vi "GenerateCode.vi"(1 "Terms":T1[](array[typedef]), 3 "Diagram":refnum<vi>, 5 "XRef":refnum<vi>, 6 "State In":T4) -> (0 "Generated Code?":bool, 2 "State Out":T4, 4 "Reply":string[](array[string]))   [LabVIEW 2012, in "Shuffle Array.xnode"]
uses:
  Shuffle Array.xnode
  State.ctl
  <vilib>/XNodeSupport/XNodeTermIDPair.ctl
  <vilib>/XNodeSupport/XNodeTermRef.ctl
  <vilib>/XNodeSupport/XNodeString.ctl
  <vilib>/Utility/miscctls.llb/LVPositionTypeDef.ctl
  <userlib>/_LAVAcr/Scripting Tools/Scripting Tools.lvlib
  <vilib>/XNodeSupport/NI_XNodeSupport.lvlib
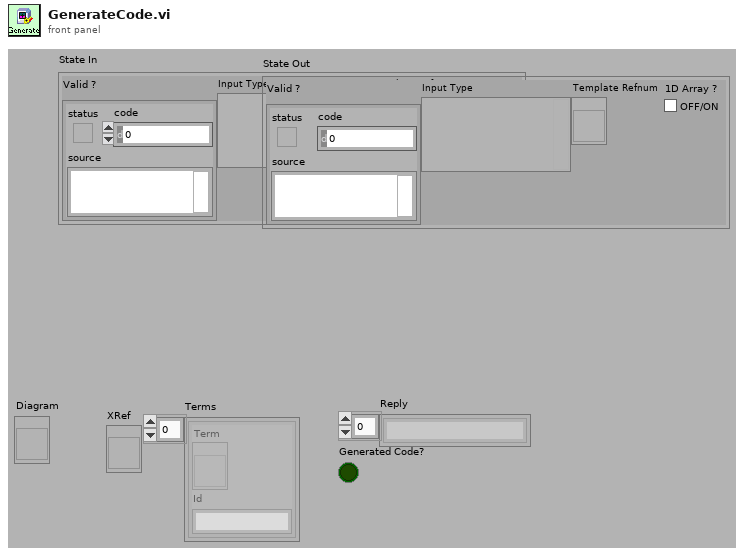
[diagram p1: front panel]
types:
  T1 = typedef "NI_XNodeSupport.lvlib/XNodeTermIDPair.ctl" = cluster{"Term":T2, "Id":T3}
  T2 = typedef "NI_XNodeSupport.lvlib/XNodeTermRef.ctl" = refnum<vi>
  T3 = typedef "NI_XNodeSupport.lvlib/XNodeString.ctl" = string
  T4 = typedef "Shuffle Array.xnode/State.ctl" = cluster{"Valid ?":errorcluster, "Input Type":variant, "Template Refnum":refnum<vi>, "1D Array ?":bool}
  T5 = typedef "LVPositionTypeDef.ctl" = cluster{"Left":i32, "Top":i32}
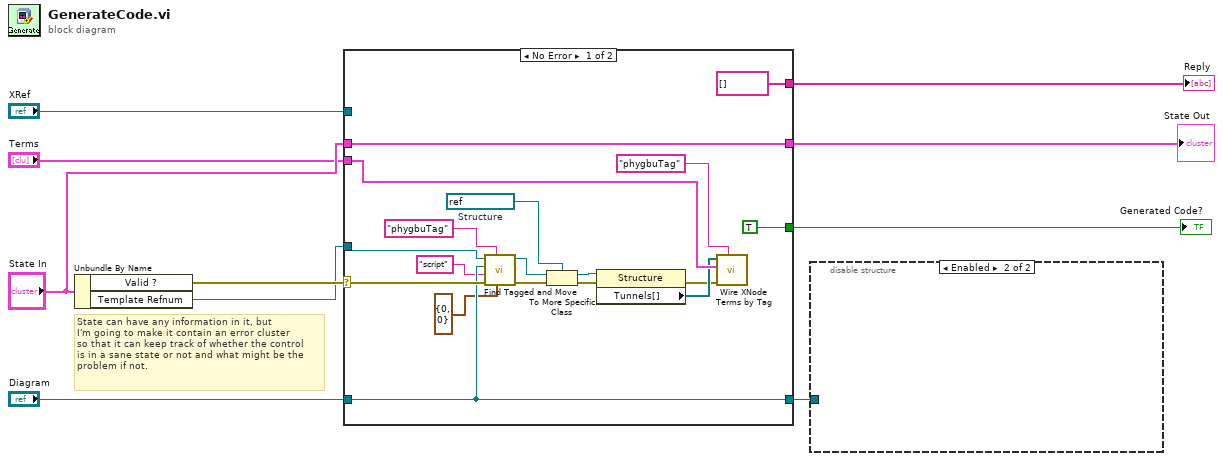
[diagram p0: block diagram]
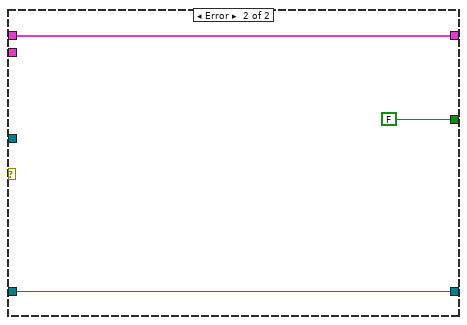
[diagram p2: hidden frame]
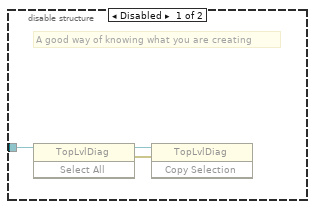
[diagram p3: hidden frame]
diagram:
  # "State can have any information in it, but\nI'm going to make it contain an error cluster\nso that it can keep track of whether the control\nis in a sane state or not and what might be the\nproblem if not."
  n1 = Unbundle By Name("State In") -> ("Valid ?"=w10:errorcluster, "Template Refnum"=w1:refnum<vi>)
  n2 = case shown="No Error" w10 {
    selector: w10 -> [w21 _]
    tunnel: "State In" -> [w26 w31]
    tunnel: "Diagram" -> [w20 w29]
    tunnel: "Terms" -> [w25 _]
    tunnel: "XRef" -> [_ _]
    tunnel: [w20 w29] -> w2
    tunnel: [string[] [] ("Reply") _] -> w5
    tunnel: [TRUE FALSE] -> w4
    tunnel: [w26 w31] -> w3
    tunnel: w1 -> [w11 _]
    frame No Error {
      w23 = refnum<vi> refnum  # Structure
      n3 = call <userlib>:"Find Tagged and Move.vi"("position"=T5 {"Left"=0, "Top"=0}, "TagName"="phygbuTag", "error in"=w21, "TagValue"="script", "Destination Diagram"=w20, "VI Refnum"=w11) -> ("error out"=w15:errorcluster, "Moved Tagged object"=w16:refnum<vi>)  [unwired: 4 out]
      n4 = To More Specific Class(target class=w23, reference=w16, error in=w15) -> (specific class reference=w24:refnum<vi>, error out=w14:errorcluster)
      n5 = property class="Structure"(reference=w24, error in=w14) -> (error out=w13:errorcluster, "Tunnels[]"=w22:refnum<vi>[])  [unwired: 1 out]
      n6 = call <userlib>:"Wire XNode Terms by Tag.vi"("TagName"="phygbuTag", "error in (no error)"=w13, "Term Refs"=w25, "Source References"=w22) -> ()  [unwired: 8 out]
    }
    frame Error {
    }
  }
  "State Out" <- w3
  "Reply" <- w5
  "Generated Code?" <- w4
  n7 = disable-structure shown="Enabled" {
    disable-tunnel: w2 -> [w32 _]
    frame Disabled {
      # "A good way of knowing what you are creating"
      n8 = invoke class="TopLvlDiag" method="Select All"(reference=w32) -> (reference out=w34:refnum<vi>, error out=w33:errorcluster)  [unwired: 2 in, 1 out]
      n9 = invoke class="TopLvlDiag" method="Copy Selection"(reference=w34, error in=w33) -> ()  [unwired: 1 in, 3 out]
    }
    frame Enabled {
    }
  }
